vi "Global-Delete System.vi"(11 "VISA session":refnum<visa-resource-name>) -> (2 "found":bool, 3 "VISA resource name out":refnum<visa-resource-name>)   [LabVIEW 2016, in "Agilent 415X Series.lvlib"]
doc: "This VI uses an instrument's \"instrument handler\" as a key to search the global system configuration table for the instrument. If the instrument is found in the table, the entry is marked \"invalid\" so\nit can be re-used by other instruments.\n\nTypical use of this VI: when closing an instrument."
uses:
  Agilent 415X Series.lvlib
  Private/Global.vi
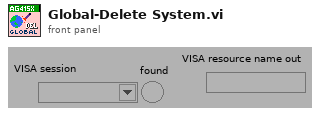
[diagram p1: front panel]
types:
  T1 = cluster{"valid instrument":bool, "GNDU present":bool, "SMU5 present":bool, "SMU6 present":bool, "PGU1 present":bool, "PGU2 present":bool, "active error checking":bool, "instr. handler":refnum<visa-resource-name>}[]
  T2 = cluster{bool, bool, bool, bool, bool, bool, bool, "instr. handler":refnum<visa-resource-name>}
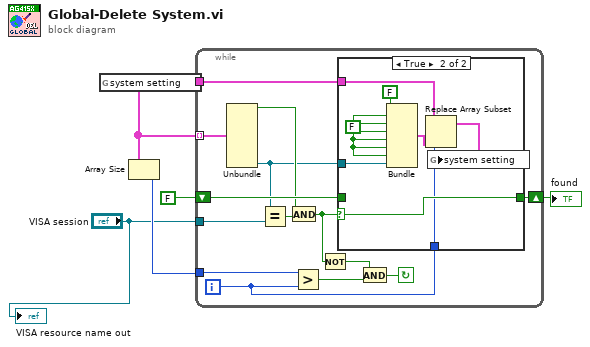
[diagram p0: block diagram]
diagram:
  n1 = global read "Global.vi" "system setting"() -> (w2:T1)
  n2 = Array Size(array=w2) -> (size(s)=w4:i32)
  n3 = while {
    tunnel: "VISA session" -> [w6]
    tunnel: w2 -> [w9]
    shift-left: FALSE -> [w12]
    shift-right: [w11] -> w3
    tunnel: w4 -> [w17]
    tunnel: w2 -> [w19] mode=indexing
    i -> [w8]
    stop <- w15 continue-if-true
    n4 = Unbundle(w19) -> ("valid instrument"=w10:bool, "instr. handler"=w7:refnum<visa-resource-name>)  [unwired: 6 out]
    n5 = Equal?(x=w7, y=w6) -> (x = y?=w18:bool)
    n6 = And(x=w10, y=w18) -> (x .and. y?=w13:bool)
    n7 = Greater?(x=w17, y=w8) -> (0:w16:bool)
    n8 = Not(x=w13) -> (.not. x?=w14:bool)
    n9 = case shown="True" w13 {
      selector: w13 -> [_ w28]
      tunnel: w12 -> [w20 _]
      tunnel: [w20 w28] -> w11
      tunnel: w9 -> [_ w25]
      tunnel: w8 -> [_ w26]
      tunnel: w7 -> [_ w22]
      frame False {
      }
      frame True {
        w21 = FALSE
        n10 = Bundle(FALSE, w21, w21, w21, w21, w21, w21, "instr. handler"=w22) -> (w23:T2)  [unwired: 1 in]
        n11 = Replace Array Subset(array=w25, new element=w23, index=w26) -> (w24:T1)
        n12 = global write "Global.vi" "system setting"(w24) -> ()
      }
    }
    n13 = And(x=w14, y=w16) -> (x .and. y?=w15:bool)
  }
  "found" <- w3
  "VISA resource name out" <- "VISA session"
